vi "Create Engine Stream Refs.vi"(4 "FD ISO Mode":u32(ring) items=["ISO", "Non ISO", "ISO Legacy"], 6 "Termination":u32(ring) items=["Off", "On"], 7 "Default IDs":u32[](array[numeric]), 8 "error in (no error)":errorcluster, 9 "Cluster":refnum<k21>, 10 "Port":refnum<k21>, 11 "Addon":string) -> (0 "error out":errorcluster, 3 "Refs":T1 {"FD ISO Mode" items=["ISO", "Non ISO", "ISO Legacy"]; "Termination" items=["Off", "On"]})   [LabVIEW 2019, in "CAN Stream Support Engine.lvlib"]
uses:
  CAN Stream Support Engine.lvlib
  Types/Engine Stream Refs.ctl
  Addon Shared/Types/Direction Filter.ctl
  Addon Shared/Types/Type Filter.ctl
  Addon Shared/Types/Filter Parameters.ctl
  Addon Shared/CAN Stream Support Shared.lvlib
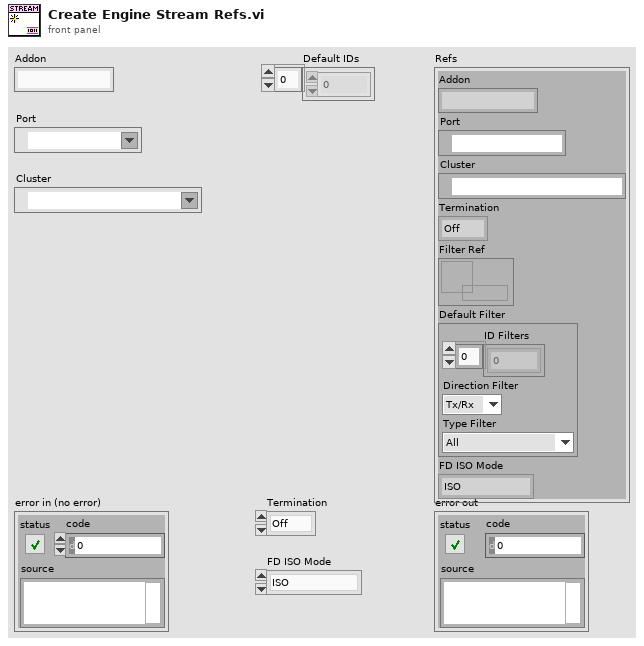
[diagram p1: front panel]
types:
  T1 = typedef "CAN Stream Support Engine.lvlib/Engine Stream Refs.ctl" = cluster{"Addon":string, "Port":refnum<k21>, "Cluster":refnum<k21>, "Termination":u32, "Filter Ref":refnum<data-value>, "Default Filter":T2, "FD ISO Mode":u32}
  T2 = typedef "CAN Stream Support Shared.lvlib/Filter Parameters.ctl" = cluster{"ID Filters":u32[], "Direction Filter":T3, "Type Filter":T4}
  T3 = typedef "CAN Stream Support Shared.lvlib/Direction Filter.ctl" = enum16{"Tx/Rx", "Rx", "Tx"}
  T4 = typedef "CAN Stream Support Shared.lvlib/Type Filter.ctl" = enum16{"All", "CAN Data", "CAN Remote", "CAN Bus Error", "CAN 2.0 Data", "CAN FD Data", "CAN FD+BRS Data", "J1939 Data", "Delay", "Log Trigger", "Start Trigger"}
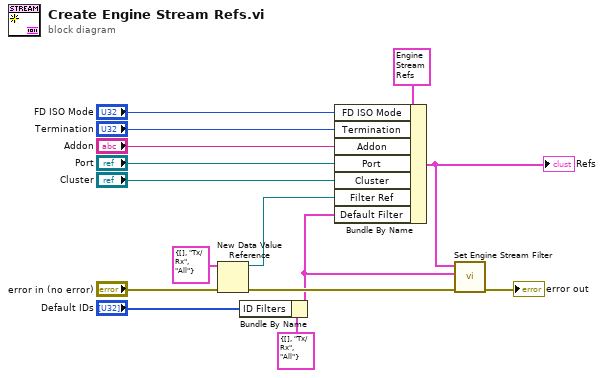
[diagram p0: block diagram]
diagram:
  n1 = New Data Value Reference(data value=T2 {"ID Filters"=[], "Direction Filter"=enum."Tx/Rx", "Type Filter"=enum."All"}, error in="error in (no error)") -> (data value reference=w5:refnum<data-value>, error out=w8:errorcluster)
  n2 = Bundle By Name(cluster=T2 {"ID Filters"=[], "Direction Filter"=enum."Tx/Rx", "Type Filter"=enum."All"} ("Filter"), "ID Filters"="Default IDs") -> (w2:T2)
  n3 = Bundle By Name(cluster=T1 {"Addon"="", "Port"="", "Cluster"="", "Termination"=0, "Filter Ref"=refnum, "Default Filter"={"ID Filters"=[], "Direction Filter"=enum."Tx/Rx", "Type Filter"=enum."All"}, "FD ISO Mode"=0}, "FD ISO Mode"="FD ISO Mode", "Termination"="Termination", "Addon"="Addon", "Port"="Port", "Cluster"="Cluster", "Filter Ref"=w5, "Default Filter"=w2) -> (w9:T1)
  "Refs" <- w9
  n4 = call "Set Engine Stream Filter.vi"("error in (no error)"=w8, "Filter"=w2, "Refs"=w9) -> ("error out"=→"error out":errorcluster)  [unwired: 8 in]
